vi "test_parse_single_param.vi"(8 "error out 2":errorcluster) -> (0 "error out":errorcluster)   [LabVIEW 2023, in "Easy.SequenceManager.Test.lvlib"]
uses:
  src/Parameter/Parameter.lvclass
  <vilib>/addons/_JKI Toolkits/Caraya/classes/Assert/Assert Equal Value and Type_Variant.vi
  Easy.SequenceManager.Test.lvlib
  <vilib>/addons/_JKI Toolkits/Caraya/classes/Test/Test.lvclass
  <vilib>/addons/_JKI Toolkits/Caraya/classes/Assert/Assert.lvclass
  <vilib>/addons/_JKI Toolkits/Caraya/classes/Assert/Assert Not Error.vi
panel:
  out "HooverOverInfo":string
  # "Connector Pane"
  # "Locals"
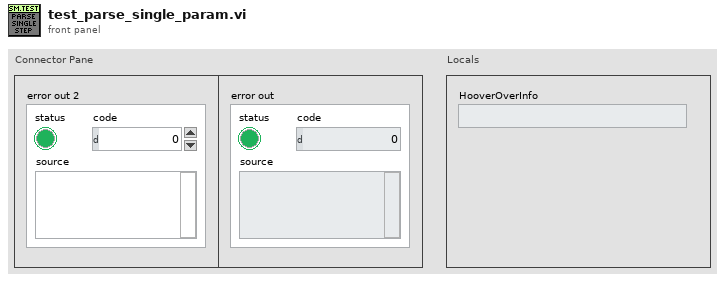
[diagram p1: front panel]
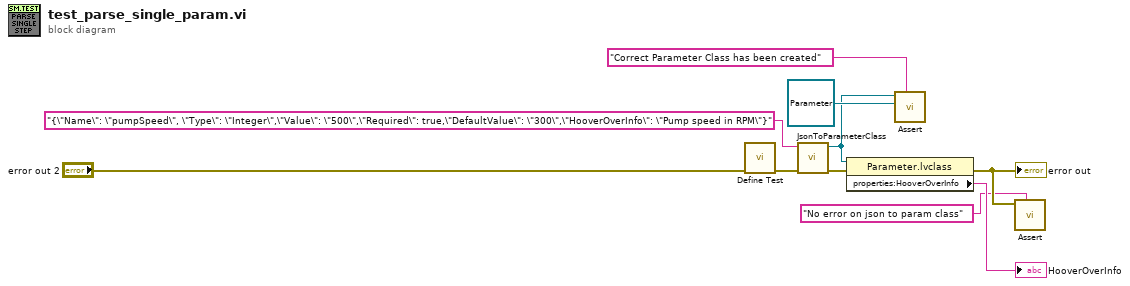
[diagram p0: block diagram]
diagram:
  n1 = call <vilib>:"Define Test.vi"("error in (no error)"="error out 2") -> ("error out"=w4:errorcluster)  [unwired: 9 in, 1 out]
  n2 = call "JsonToParameterClass.vi"("error in (no error)"=w4, "JSON String"="{\"Name\": \"pumpSpeed\", \"Type\": \"Integer\",\"Value\": \"500\",\"Required\": true,\"DefaultValue\": \"300\",\"HooverOverInfo\": \"Pump speed in RPM\"}") -> ("error out"=w3:errorcluster, "Parameter Out"=w7:refnum<class "Parameter.lvclass">)  [unwired: 8 in]
  n3 = property class="Parameter.lvclass"(reference=w7, error in=w3) -> (error out=w2:errorcluster, "properties:HooverOverInfo"=→"HooverOverInfo":string)  [unwired: 1 out]
  "error out" <- w2
  n4 = call-poly <vilib>:"Assert.vi"("Label"="Correct Parameter Class has been created" ("Label (VI Title)"), "Y"=refnum<class "Parameter.lvclass"> refnum ("Parameter Out"), "X"=w7) -> ()  [unwired: 7 in, 2 out]
  n5 = call-poly <vilib>:"Assert.vi"("Label"="No error on json to param class", "Not Error?"=w2) -> ()  [unwired: 8 in, 2 out]
